vi "Read Video Frames.vi"(9 "frame":i32, 10 "Path":path, 11 "Refnum in":T1) -> (2 "Number of Frames":i32, 3 "Refnum out":T1)   [LabVIEW 2019]
uses:
  <vilib>/vision/Image Controls.llb/IMAQ Image.ctl
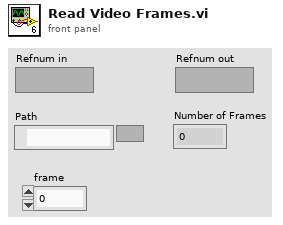
[diagram p1: front panel]
types:
  T1 = typedef "IMAQ Image.ctl" = refnum<image>
  T2 = typedef "IMAQ AVI2 Refnum.ctl" = refnum<k20>
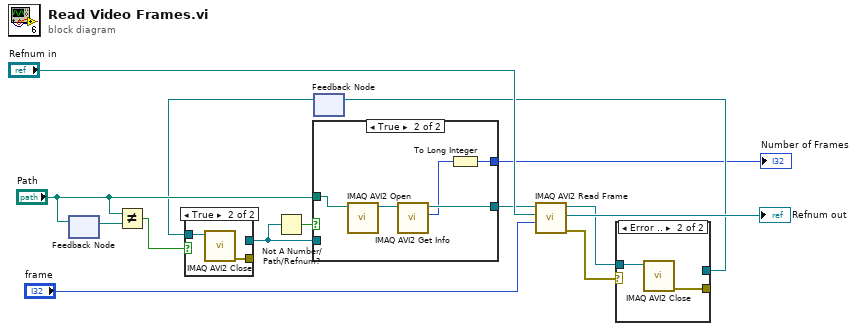
[diagram p0: block diagram]
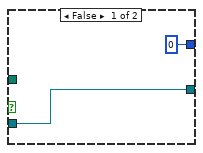
[diagram p4: hidden frame]
diagram:
  n1 = feedback #1() -> (w5:path)  [unwired: 1 in]
  n2 = feedback-in #1("Path") -> ()
  n3 = Not Equal?(x="Path", y=w5) -> (x != y?=w3:bool)
  n4 = feedback #2() -> (w2:T2)  [unwired: 1 in]
  n5 = case shown="True" w3 {
    tunnel: w2 -> [w15 w17]
    tunnel: [w15 _] -> w1
    tunnel: [_ w16] -> _
    frame False {
    }
    frame True {
      n6 = call "IMAQ AVI2 Close"("AVI Refnum"=w17) -> ("error out"=w16:errorcluster)  [unwired: 10 in]
    }
  }
  n7 = Not A Number/Path/Refnum?(number/path/refnum=w1) -> (NaN/Path/Refnum?=w10:bool)
  n8 = case shown="True" w10 {
    tunnel: [w19 w22] -> w11
    tunnel: w1 -> [w19 _]
    tunnel: "Path" -> [_ w24]
    tunnel: [0 ("Number of Frames") w20] -> w7
    frame False {
    }
    frame True {
      n9 = call "IMAQ AVI2 Open"("AVI File Path"=w24) -> ("AVI Refnum"=w23:T2)  [unwired: 9 in, 1 out]
      n10 = call "IMAQ AVI2 Get Info"("AVI Refnum"=w23) -> ("Number of Frames"=w21:u32, "AVI Refnum (duplicate)"=w22:T2)  [unwired: 6 in, 3 out]
      n11 = To Long Integer(number=w21) -> (32bit integer=w20:i32)
    }
  }
  "Number of Frames" <- w7
  n12 = call "IMAQ AVI2 Read Frame"("Frame Number"="frame", "Image"="Refnum in", "AVI Refnum"=w11) -> ("error out"=w14:errorcluster, "Image Out"=→"Refnum out":T1, "AVI Refnum (duplicate)"=w9:T2)  [unwired: 6 in]
  n13 = case shown="Error .." w14 {
    tunnel: w9 -> [w25 w27]
    tunnel: [w25 _] -> w8
    tunnel: [_ w26] -> _
    frame No Error {
    }
    frame Error {
      n14 = call "IMAQ AVI2 Close"("AVI Refnum"=w27) -> ("error out"=w26:errorcluster)  [unwired: 10 in]
    }
  }
  n15 = feedback-in #2(w8) -> ()
